vi "Chroma 1905x Series Configure w492 h337 1.vi"(7 "Mode":T1 items=["DC", "IR"], 8 "error in (no error)":errorcluster, 9 "Dwell Time [s]":dbl min=0.0 max=999.0 step=0.1 format="%.3p", 10 "Step":u8=1 min=1 max=99 step=1, 11 "VISA resource name":refnum<visa-resource-name>) -> (0 "error out":errorcluster, 3 "VISA resource name out":refnum<visa-resource-name>)   [LabVIEW 2025]
uses:
  <instrlib>/Chroma 19052/Chroma 19052.lvlib
  <instrlib>/Chroma 19052/Public/Utility/Type Def/DC-IR modes--ring.ctl
panel:
  # "Configure Dwell Time"
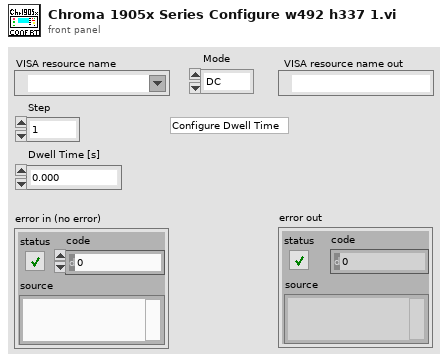
[diagram p1: front panel]
types:
  T1 = typedef "DC-IR modes--ring.ctl" = u16
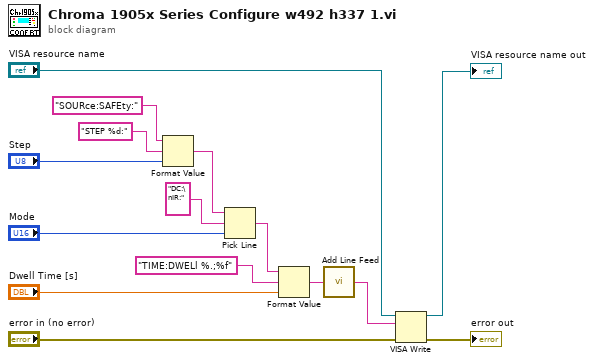
[diagram p0: block diagram]
diagram:
  n1 = Format Value(string ("")="SOURce:SAFEty:", format string="STEP %d:", value (0)="Step") -> (output string=w10:string)
  n2 = Pick Line(string ("")=w10, multi-line string="DC:\nIR:", line index="Mode") -> (output string=w8:string)
  n3 = Format Value(string ("")=w8, format string="TIME:DWELl %.;%f", value (0)="Dwell Time [s]") -> (output string=w6:string)
  n4 = call <instrlib>:"Add Line Feed.vi"("Command string"=w6) -> ("Concatenated string"=w5:string)  [unwired: 4 in]
  n5 = VISA Write(VISA resource name="VISA resource name", write buffer=w5, error in (no error)="error in (no error)") -> (VISA resource name out=→"VISA resource name out":refnum<visa-resource-name>, error out=→"error out":errorcluster)  [unwired: 1 out]
